vi "DriveForwardAuton.vi"(11 "Milliseconds (Default to 1200)":dbl=1200.0) -> ()   [LabVIEW 2013]
uses:
  <vilib>/Rock Robotics/WPI/SafetyOutput/WPI_SafetyOutputConfigMenu.ctl
  <vilib>/Rock Robotics/WPI/RobotDrive/WPI_RobotDriveGetSetRefNum.vi
  <vilib>/Rock Robotics/WPI/RobotDrive/WPI_RobotDriveArcadeDrive_Standard(NoSaturation).vi
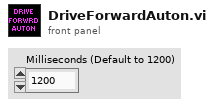
[diagram p1: front panel]
types:
  T1 = typedef "WPI_SafetyOutputConfigMenu.ctl" = enum16{"Enable", "Disable"}
  T2 = typedef "WPI_RobotDriveDevRef.ctl" = cluster{"DevStatus":errorcluster, "Motors[]":T3[], "Square Inputs":bool, "Max Output":dbl, "Isochronous":bool}
  T3 = typedef "WPI_MotorControlDeviceRef.ctl" = cluster{"DeviceStatus":errorcluster, "Type":enum16{"PWM", "CAN"}, "PWM":cluster{"Digital Module":T4, "PWM Channel":T5, "DeadBand":T6}, "CAN":cluster{"Device Number":u8, "Control Mode":T7, "Semaphore":T8, "Max Vout":dbl}, "Invert":bool, "TransformRef":T9, "InvTransformRef":T9}
  T4 = typedef "FPGA_TypedefDigitalModule.ctl" = enum16{"Digital Module 1", "Digital Module 2"}
  T5 = typedef "FPGA_DIOPWMChannel.ctl" = enum8{"PWM 1", "PWM 2", "PWM 3", "PWM 4", "PWM 5", "PWM 6", "PWM 7", "PWM 8", "PWM 9", "PWM 10", "Invalid"}
  T6 = typedef "WPI_PWMDeadband.ctl" = cluster{"Name":string, "maxPositivePwm":i32, "minPositivePwm":i32, "centerPwm":i32, "maxNegativePwm":i32, "minNegativePwm":i32, "angularRange":u16}
  T7 = typedef "WPI_CANJaguar_ControlMode.ctl" = enum8{"Percent VBus", "Current", "Speed", "Position", "Voltage"}
  T8 = typedef "Semaphore RefNum" = refnum<k1>
  T9 = typedef "WPI_PWMTransform_ConPane.ctl" = refnum<vi>
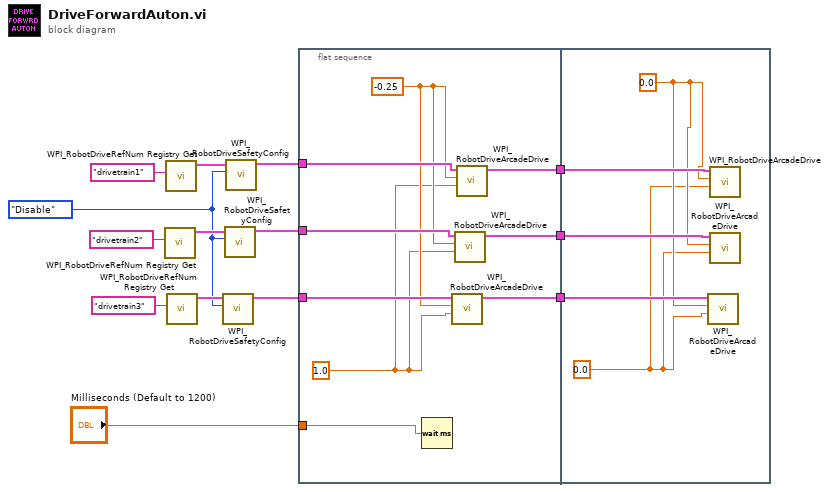
[diagram p0: block diagram]
diagram:
  w8 = WPI_SafetyOutputConfigMenu."Disable" ("mode")
  n1 = call <vilib>:"WPI_RobotDriveRefNum Registry Get.vi"("refnum name"="drivetrain2") -> ("RobotDriveDevRef"=w10:T2)  [unwired: 9 in, 1 out]
  n2 = call <vilib>:"WPI_RobotDriveRefNum Registry Get.vi"("refnum name"="drivetrain1") -> ("RobotDriveDevRef"=w11:T2)  [unwired: 9 in, 1 out]
  n3 = call <vilib>:"WPI_RobotDriveRefNum Registry Get.vi"("refnum name"="drivetrain3") -> ("RobotDriveDevRef"=w9:T2)  [unwired: 9 in, 1 out]
  n4 = call <vilib>:"WPI_RobotDriveSafetyConfig.vi"("mode"=w8, "RobotDriveDevRef"=w9) -> ("RobotDriveDevRef"=w5:T2)  [unwired: 8 in, 1 out]
  n5 = call <vilib>:"WPI_RobotDriveSafetyConfig.vi"("mode"=w8, "RobotDriveDevRef"=w10) -> ("RobotDriveDevRef"=w6:T2)  [unwired: 8 in, 1 out]
  n6 = call <vilib>:"WPI_RobotDriveSafetyConfig.vi"("mode"=w8, "RobotDriveDevRef"=w11) -> ("RobotDriveDevRef"=w7:T2)  [unwired: 8 in, 1 out]
  n7 = flat-sequence {
    tunnel: w7 -> [w23]
    tunnel: w6 -> [w22]
    tunnel: w5 -> [w21]
    tunnel: [w18] -> w4
    tunnel: [w17] -> w3
    tunnel: [w16] -> w2
    tunnel: "Milliseconds (Default to 1200)" -> [w15]
    tunnel: w4 -> [w28]
    tunnel: w3 -> [w27]
    tunnel: w2 -> [w26]
    frame #0 {
      w19 = 1.0 ("Y axis value")
      w20 = -0.25 ("X axis value")
      n8 = Wait (ms)(milliseconds to wait=w15) -> ()  [unwired: 1 out]
      n9 = call-poly <vilib>:"WPI_RobotDriveArcadeDrive.vi"("Y axis value"=w19, "X axis value"=w20, "RobotDriveDevRef"=w21) -> ("RobotDriveDevRef"=w18:T2)  [unwired: 6 in, 2 out]
      n10 = call-poly <vilib>:"WPI_RobotDriveArcadeDrive.vi"("Y axis value"=w19, "X axis value"=w20, "RobotDriveDevRef"=w22) -> ("RobotDriveDevRef"=w17:T2)  [unwired: 6 in, 2 out]
      n11 = call-poly <vilib>:"WPI_RobotDriveArcadeDrive.vi"("Y axis value"=w19, "X axis value"=w20, "RobotDriveDevRef"=w23) -> ("RobotDriveDevRef"=w16:T2)  [unwired: 6 in, 2 out]
    }
    frame #1 {
      w24 = 0.0 ("X axis value")
      w25 = 0.0 ("X axis value")
      n12 = call-poly <vilib>:"WPI_RobotDriveArcadeDrive.vi"("Y axis value"=w24, "X axis value"=w25, "RobotDriveDevRef"=w28) -> ()  [unwired: 6 in, 3 out]
      n13 = call-poly <vilib>:"WPI_RobotDriveArcadeDrive.vi"("Y axis value"=w24, "X axis value"=w25, "RobotDriveDevRef"=w26) -> ()  [unwired: 6 in, 3 out]
      n14 = call-poly <vilib>:"WPI_RobotDriveArcadeDrive.vi"("Y axis value"=w24, "X axis value"=w25, "RobotDriveDevRef"=w27) -> ()  [unwired: 6 in, 3 out]
    }
  }
